vi "Write Camera Setup.vi"(8 "error in (no error)":errorcluster, 10 "RED Channel Settings":T1={"Cooler ON/OFF"=0, "Set temperature"=20.0, "Temperature ºC"=0.0, "Shutter Mode "=2, "Shutter TTL"=0, "Time to open (ms)"=50.0, "Time to close (ms)"=50.0, "Baseline Clamp 2"=FALSE, "EM Advanced 2"=FALSE, "EM Gain  level "=1, "EM Gain"=FALSE, "Pre-amplifier gain"=1, "Vertical clock\n  voltage amplitude"=0, "Vertical Shift Speed"=0, "Readout Rate "=0, "Trigger "=0, "Conventional/EM"=1, "Read Mode "=4, "Acquisition Mode "=1, "Exposure Time (s) "=0.0, "XY Graph"=[], "Sub Image"=enum."1024 x 1024", "Initial Line"=1, "Initial Column"=1, "Final Line"=1, "Final Column"=1, "Horizontal binning"=1, "Vertical binning "=1, "# Exposure"=1, "Image Name"="", "Night Directory"="", "FITS Format"=0, "Image Format"="", "Tiff Position "=1, "Tiff Type"=0} {"Tiff Type" items=["8-bit", "16-bit", "Color"]; "FITS Format" items=["Unsigned 16", "Unsigned 32", "Signed 16", "Signed 32", "Float"]; "# Exposure" min=1; "Exposure Time (s)" format="%.2f"; "Acquisition Mode" items=["RESERVED", "Single Scan", "Accumulate", "Kinetics", "Fast Kinetics", "Run Til Abort", "RESERVED", "RESERVED", "RESERVED", "RESERVED", "Time Delayed Integration"]; "Read Mode" items=["Full Vertical Binning", "Multi-Track", "Random-Track", "Single-Track", "Image"]; "Conventional/EM" items=["EM Gain", "Conventional"]; "Trigger" items=["Internal", "External", "N/A", "N/A", "N/A", "N/A", "External Start", "External Exposure (bulb)", "N/A", "External FVB EM", "Software", "N/A", "External Charge Shifting"]; "Shutter TTL" items=["TTL Low", "TTL High"]; "Shutter Mode" items=["Fully Auto", "OPEN", "CLOSED"]; "Temperature ºC" scale=-100.0..30.0; "Set temperature" min=-80.0 max=20.0; "Cooler ON/OFF" items=["Cooler OFF", "Cooler ON"]}, 11 "CCDCamera in":refnum<class "CCDCamera.lvclass">) -> (0 "error out":errorcluster, 3 "CCDCamera out":refnum<class "CCDCamera.lvclass">)   [LabVIEW 2018, in "CCDCamera.lvclass"]
doc: "This VI presents an interface to setup the camera configuration. The information is write to the class."
uses:
  CCDCamera.lvclass
  CCDCamera.lvclass/CCDCamera.ctl
panel:
  # "Set Shutter Configuration"
  # "Timings"
  # "Vertical pixel shift"
  # "(TTL level required to open \nyour external shutter)"
  # "Time to open/close shutter"
  # "Horizontal pixel shift"
  # "Temperature"
  # "Electron Multiplier (EM) Gain"
  # "Baseline"
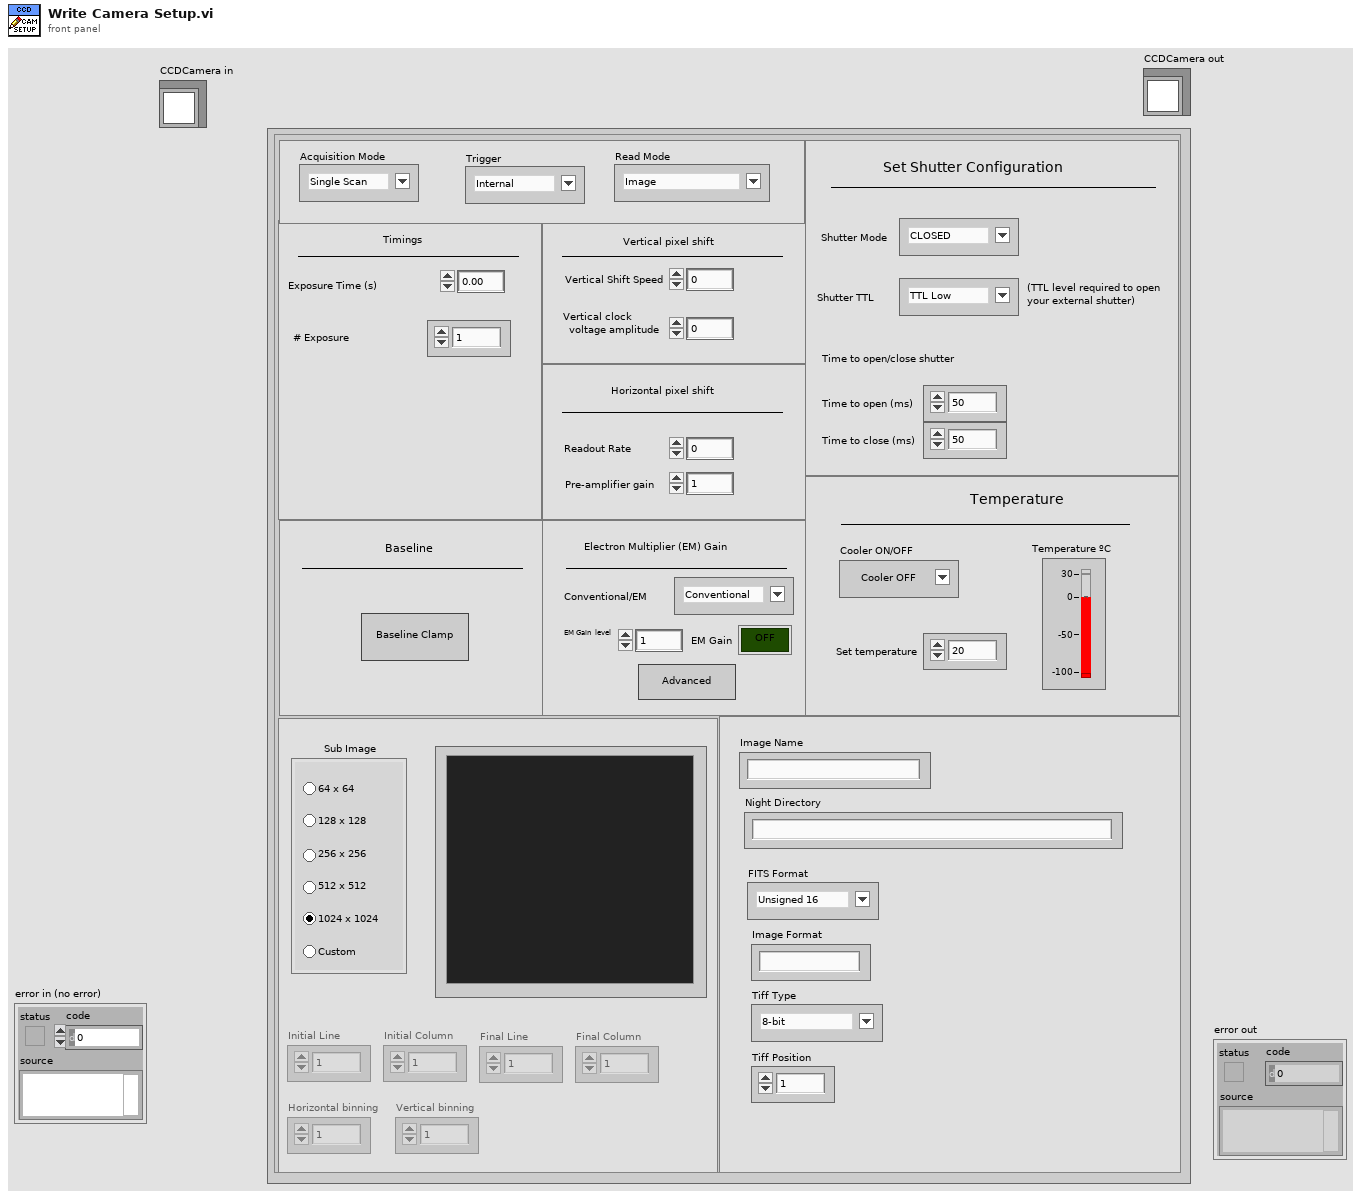
[diagram p1: front panel]
types:
  T1 = cluster{"Cooler ON/OFF":u16, "Set temperature":dbl, "Temperature ºC":dbl, "Shutter Mode ":u16, "Shutter TTL":u16, "Time to open (ms)":dbl, "Time to close (ms)":dbl, "Baseline Clamp 2":bool, "EM Advanced 2":bool, "EM Gain  level ":i32, "EM Gain":bool, "Pre-amplifier gain":i32, "Vertical clock\n  voltage amplitude":i32, "Vertical Shift Speed":i32, "Readout Rate ":i32, "Trigger ":u16, "Conventional/EM":i32, "Read Mode ":u16, "Acquisition Mode ":u16, "Exposure Time (s) ":sgl, "XY Graph":cluster{dbl, dbl}[], "Sub Image":enum32{"256 x 256", "512 x 512", "1024 x 1024", "Custom", "128 x 128", "64 x 64"}, "Initial Line":i32, "Initial Column":i32, "Final Line":i32, "Final Column":i32, "Horizontal binning":i32, "Vertical binning ":i32, "# Exposure":u32, "Image Name":string, "Night Directory":string, "FITS Format":u16, "Image Format":string, "Tiff Position ":u16, "Tiff Type":u16}
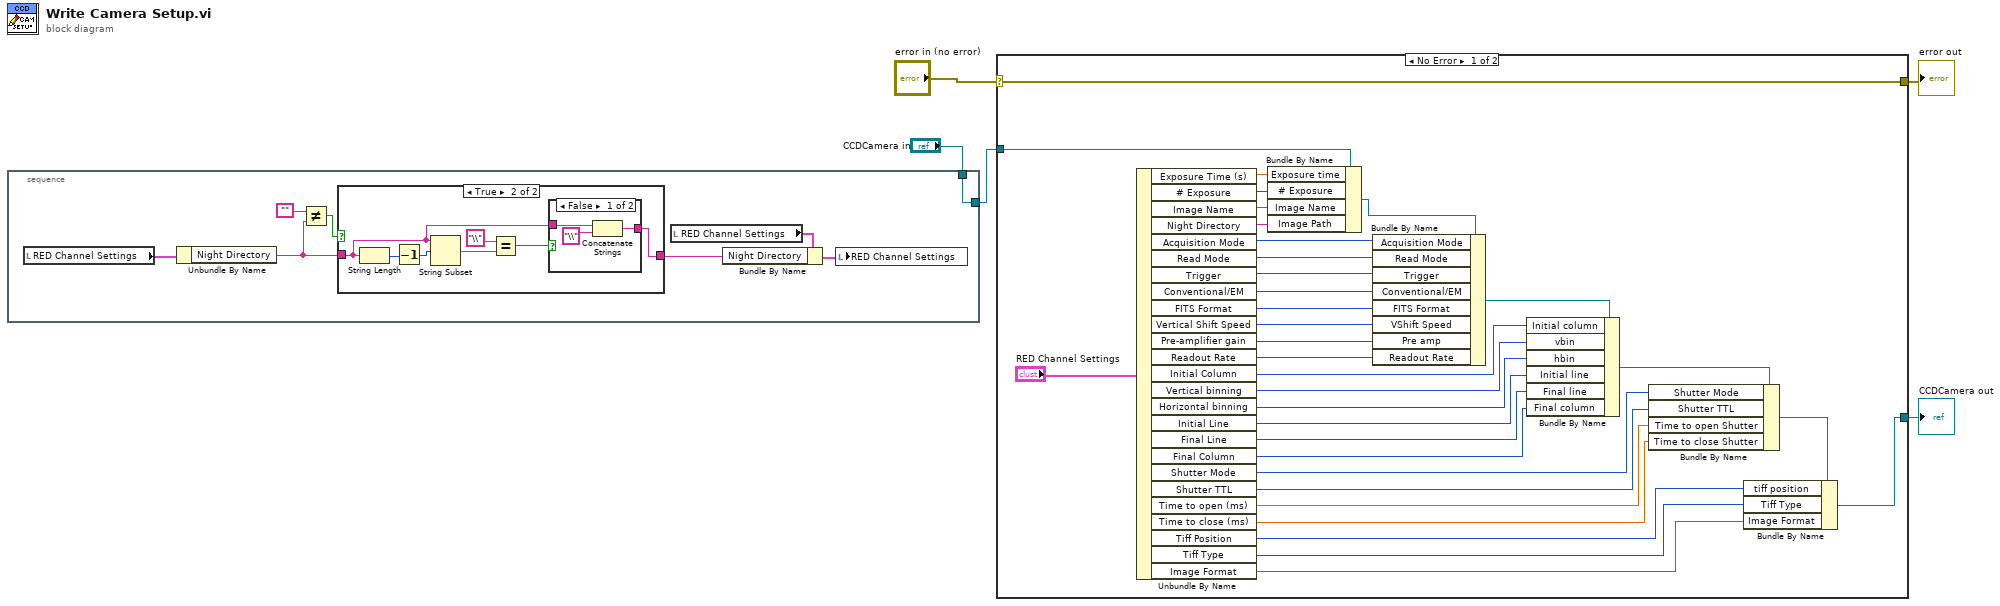
[diagram p0: block diagram]
diagram:
  n1 = stacked-sequence {
    tunnel: "CCDCamera in" -> [w9]
    tunnel: [w9] -> w1
    frame #0 {
      n2 = local read "RED Channel Settings"() -> (w13:T1)
      n3 = Unbundle By Name(w13) -> ("Night Directory"=w7:string)
      n4 = Not Equal?(x="", y=w7) -> (x != y?=w8:bool)
      n5 = case shown="True" w8 {
        tunnel: w7 -> [w14 w16]
        tunnel: [w14 w15] -> w12
        frame False {
        }
        frame True {
          n6 = String Length(string=w16) -> (length=w21:i32)
          n7 = Decrement(x=w21) -> (x-1=w20:i32)
          n8 = String Subset(string=w16, offset (0)=w20) -> (substring=w19:string)  [unwired: 1 in]
          n9 = Equal?(x="\\", y=w19) -> (x = y?=w17:bool)
          n10 = case shown="False" w17 {
            tunnel: w16 -> [w24 w25]
            tunnel: [w22 w25] -> w15
            frame False {
              n11 = Concatenate Strings(w24, "\\" ("x")) -> (w22:string)
            }
            frame True {
            }
          }
        }
      }
      n12 = local read "RED Channel Settings"() -> (w11:T1)
      n13 = Bundle By Name(cluster=w11, "Night Directory"=w12) -> (w10:T1)
      n14 = local write "RED Channel Settings"(w10) -> ()
    }
  }
  n15 = case shown="No Error" "error in (no error)" {
    selector: "error in (no error)" -> [w58 w60]
    tunnel: [w58 w60] -> w4
    tunnel: [w29 w59] -> w3
    tunnel: w1 -> [w35 w59]
    frame No Error {
      n16 = Unbundle By Name("RED Channel Settings") -> ("Exposure Time (s)"=w37:sgl, "# Exposure"=w38:u32, "Image Name"=w39:string, "Night Directory"=w40:string, "Acquisition Mode"=w41:u16, "Read Mode"=w42:u16, "Trigger"=w43:u16, "Conventional/EM"=w44:i32, "FITS Format"=w45:u16, "Vertical Shift Speed"=w46:i32, "Pre-amplifier gain"=w47:i32, "Readout Rate"=w48:i32, "Initial Column"=w49:i32, "Vertical binning"=w50:i32, "Horizontal binning"=w51:i32, "Initial Line"=w52:i32, "Final Line"=w53:i32, "Final Column"=w54:i32, "Shutter Mode"=w55:u16, "Shutter TTL"=w56:u16, "Time to open (ms)"=w57:dbl, "Time to close (ms)"=w31:dbl, "Tiff Position"=w28:u16, "Tiff Type"=w27:u16, "Image Format"=w26:string)
      n17 = Bundle By Name(cluster=w35, "Exposure time"=w37, "# Exposure"=w38, "Image Name"=w39, "Image Path"=w40) -> (w34:refnum<class "CCDCamera.lvclass">)
      n18 = Bundle By Name(cluster=w34, "Acquisition Mode"=w41, "Read Mode"=w42, "Trigger"=w43, "Conventional/EM"=w44, "FITS Format"=w45, "VShift Speed"=w46, "Pre amp"=w47, "Readout Rate"=w48) -> (w33:refnum<class "CCDCamera.lvclass">)
      n19 = Bundle By Name(cluster=w33, "Initial column"=w49, "vbin"=w50, "hbin"=w51, "Initial line"=w52, "Final line"=w53, "Final column"=w54) -> (w32:refnum<class "CCDCamera.lvclass">)
      n20 = Bundle By Name(cluster=w32, "Shutter Mode"=w55, "Shutter TTL"=w56, "Time to open Shutter"=w57, "Time to close Shutter"=w31) -> (w30:refnum<class "CCDCamera.lvclass">)
      n21 = Bundle By Name(cluster=w30, "tiff position"=w28, "Tiff Type"=w27, "Image Format"=w26) -> (w29:refnum<class "CCDCamera.lvclass">)
    }
    frame Error {
    }
  }
  "error out" <- w4
  "CCDCamera out" <- w3
